vi "Lab Panel V6.00.vi"() -> ()   [LabVIEW 2017] (continued)
              n212 = call "sub vi-open serial port v1.vi"("Select COM port"=w223) -> ("Error"=→"Com Port Status":bool, "LOOPS"=→"Com setup loops":i32, "VISA Com out"=→"VISA Com out":refnum<visa-resource-name>)  [unwired: 12 in]
            }
            frame #1 {
              n213 = for {
                N: 1 -> [_]
                w274 = TRUE
                n214 = local read "Temp Simulate"() -> (w230:bool)
                n215 = local write "Temp read loop"(0) -> ()
                n216 = case shown="True" w230 {
                  frame False {
                  }
                  frame True {
                    w276 = 20
                    n217 = local write "Ambient Volts"(2.92) -> ()
                    n218 = global write "Global display 3.vi" "Ref deg C"(w276) -> ()
                    n219 = local write "Ref deg C"(w276) -> ()
                  }
                }
                n220 = call "sub vi - GET ALL TEMP v7.vi"("LA01-EN"=w274, "LA02-EN"=w274, "LA03-EN"=w274, "LA04-EN"=w274, "LA05-EN"=w274, "simulate"=w230, "Gen Cal Value"=1) -> ("ID"=w236:T29, "LA01 TEMP"=w272:T30, "LA02 TEMP"=w265:T30, "LA04 TEMP"=w251:T30, "LA03 TEMP"=w258:T30, "LA05 TEMP"=w244:T30)  [unwired: 3 in, 4 out]
                n221 = local write "LAB05 TEMP"(w244) -> ()
                n222 = local write "LAB04 TEMP"(w251) -> ()
                n223 = Unbundle(w258) -> ("T1"=w255:dbl, "T2"=w254:dbl, "T3"=w253:dbl, "T4"=w252:dbl)  [unwired: 2 out]
                n224 = Unbundle(w272) -> ("T1"=w270:dbl, "T2"=w269:dbl, "T3"=w268:dbl, "T4"=w267:dbl)  [unwired: 2 out]
                n225 = Unbundle(w265) -> ("T1"=w262:dbl, "T2"=w261:dbl, "T3"=w260:dbl, "T4"=w259:dbl)  [unwired: 2 out]
                n226 = Unbundle(w251) -> ("T1"=w249:dbl, "T2"=w248:dbl, "T3"=w247:dbl, "T4"=w246:dbl)  [unwired: 2 out]
                n227 = Unbundle(w244) -> ("T1"=w242:dbl, "T2"=w241:dbl, "T3"=w240:dbl, "T4"=w239:dbl)  [unwired: 2 out]
                n228 = local write "LAB01 TEMP"(w272) -> ()
                n229 = local write "LAB02 TEMP"(w265) -> ()
                n230 = local write "LAB03 TEMP"(w258) -> ()
                n231 = Unbundle(w236) -> ("id1"=→"LAB01-TP":bool, "id2"=→"LAB02-TP":bool, "id3"=→"LAB03-TP":bool, "id4"=→"LAB04-TP":bool, "id5"=→"LAB05-TP":bool)
                n232 = local read "TEMP LA05"() -> (w243:T9)
                n233 = local read "TEMP LA04"() -> (w250:T9)
                n234 = local read "TEMP LA02"() -> (w264:T9)
                n235 = local read "TEMP LA03"() -> (w257:T9)
                n236 = local read "TEMP LA01"() -> (w271:T9)
                n237 = Bundle(cluster=w257, "TL-1"=w255, "TN-1"=w254, "TL-2"=w253, "TN-2"=w252) -> (w256:T9)  [unwired: 4 in]
                n238 = Bundle(cluster=w271, "TL-1"=w270, "TN-1"=w269, "TL-2"=w268, "TN-2"=w267) -> (w266:T9)  [unwired: 4 in]
                n239 = Bundle(cluster=w264, "TL-1"=w262, "TN-1"=w261, "TL-2"=w260, "TN-2"=w259) -> (w263:T9)  [unwired: 4 in]
                n240 = Bundle(cluster=w250, "TL-1"=w249, "TN-1"=w248, "TL-2"=w247, "TN-2"=w246) -> (w245:T9)  [unwired: 4 in]
                n241 = Bundle(cluster=w243, "TL-1"=w242, "TN-1"=w241, "TL-2"=w240, "TN-2"=w239) -> (w238:T9)  [unwired: 4 in]
                n242 = local write "TEMP LA03"(w256) -> ()
                n243 = local write "TEMP LA01"(w266) -> ()
                n244 = local write "TEMP LA02"(w263) -> ()
                n245 = local write "TEMP LA05"(w238) -> ()
                n246 = local write "TEMP LA04"(w245) -> ()
              }
            }
            frame #2 {
              w285 = 0
              n247 = local read "LAB01 TEMP"() -> (w287:T12)
              n248 = local read "SIG LAB01-2"() -> (w282:T2)
              n249 = Unbundle By Name(w287) -> ("T1 Live"=w280:dbl, "T1 Neut"=w279:dbl, "T2 Live"=w278:dbl, "T2 Neut"=w277:dbl)  [unwired: 2 out]
              n250 = local read "SIG LAB01-1"() -> (w284:T2)
              n251 = local read "TEMP LA01"() -> (w288:T9)
              n252 = Bundle By Name(cluster=w288, "TL-1"=w280, "TN-1"=w279, "TL-2"=w278, "TN-2"=w277, "TL -1COUNT"=w285, "TN-1 COUNT"=w285, "TL-2 COUNT"=w285, "TN-2 COUNT"=w285) -> (w286:T9)
              n253 = Bundle(cluster=w284, "Tmp Live"=w280, "Tmp Neut"=w279) -> (w283:T2)  [unwired: 3 in]
              n254 = Bundle(cluster=w282, "Tmp Live"=w278, "Tmp Neut"=w277) -> (w281:T2)  [unwired: 3 in]
              n255 = local write "SIG LAB01-2"(w281) -> ()
              n256 = local write "SIG LAB01-1"(w283) -> ()
              n257 = local write "TEMP LA01"(w286) -> ()
            }
            frame #3 {
              w297 = 0
              n258 = local read "LAB02 TEMP"() -> (w299:T12)
              n259 = Unbundle By Name(w299) -> ("T1 Live"=w292:dbl, "T1 Neut"=w291:dbl, "T2 Live"=w290:dbl, "T2 Neut"=w289:dbl)  [unwired: 2 out]
              n260 = local read "SIG LAB02-1"() -> (w296:T2)
              n261 = local read "SIG LAB02-2"() -> (w295:T2)
              n262 = local read "TEMP LA02"() -> (w300:T9)
              n263 = Bundle By Name(cluster=w300, "TL-1"=w292, "TN-1"=w291, "TL-2"=w290, "TN-2"=w289, "TL -1COUNT"=w297, "TN-1 COUNT"=w297, "TL-2 COUNT"=w297, "TN-2 COUNT"=w297) -> (w298:T9)
              n264 = Bundle(cluster=w295, "Tmp Live"=w290, "Tmp Neut"=w289) -> (w293:T2)  [unwired: 3 in]
              n265 = Bundle(cluster=w296, "Tmp Live"=w292, "Tmp Neut"=w291) -> (w294:T2)  [unwired: 3 in]
              n266 = local write "TEMP LA02"(w298) -> ()
              n267 = local write "SIG LAB02-1"(w294) -> ()
              n268 = local write "SIG LAB02-2"(w293) -> ()
            }
            frame #4 {
              w309 = 0
              n269 = local read "LAB03 TEMP"() -> (w311:T12)
              n270 = Unbundle By Name(w311) -> ("T1 Live"=w304:dbl, "T1 Neut"=w303:dbl, "T2 Live"=w302:dbl, "T2 Neut"=w301:dbl)  [unwired: 2 out]
              n271 = local read "SIG LAB03-1"() -> (w308:T2)
              n272 = local read "SIG LAB03-2"() -> (w307:T2)
              n273 = local read "TEMP LA03"() -> (w312:T9)
              n274 = Bundle By Name(cluster=w312, "TL-1"=w304, "TN-1"=w303, "TL-2"=w302, "TN-2"=w301, "TL -1COUNT"=w309, "TN-1 COUNT"=w309, "TL-2 COUNT"=w309, "TN-2 COUNT"=w309) -> (w310:T9)
              n275 = Bundle(cluster=w307, "Tmp Live"=w302, "Tmp Neut"=w301) -> (w305:T2)  [unwired: 3 in]
              n276 = Bundle(cluster=w308, "Tmp Live"=w304, "Tmp Neut"=w303) -> (w306:T2)  [unwired: 3 in]
              n277 = local write "TEMP LA03"(w310) -> ()
              n278 = local write "SIG LAB03-2"(w305) -> ()
              n279 = local write "SIG LAB03-1"(w306) -> ()
            }
            frame #5 {
              w321 = 0
              n280 = local read "LAB04 TEMP"() -> (w323:T12)
              n281 = Unbundle By Name(w323) -> ("T1 Live"=w316:dbl, "T1 Neut"=w315:dbl, "T2 Live"=w314:dbl, "T2 Neut"=w313:dbl)  [unwired: 2 out]
              n282 = local read "SIG LAB04-2"() -> (w319:T2)
              n283 = local read "SIG LAB04-1"() -> (w320:T2)
              n284 = local read "TEMP LA04"() -> (w324:T9)
              n285 = Bundle By Name(cluster=w324, "TL-1"=w316, "TN-1"=w315, "TL-2"=w314, "TN-2"=w313, "TL -1COUNT"=w321, "TN-1 COUNT"=w321, "TL-2 COUNT"=w321, "TN-2 COUNT"=w321) -> (w322:T9)
              n286 = Bundle(cluster=w319, "Tmp Live"=w314, "Tmp Neut"=w313) -> (w317:T2)  [unwired: 3 in]
              n287 = Bundle(cluster=w320, "Tmp Live"=w316, "Tmp Neut"=w315) -> (w318:T2)  [unwired: 3 in]
              n288 = local write "SIG LAB04-2"(w317) -> ()
              n289 = local write "TEMP LA04"(w322) -> ()
              n290 = local write "SIG LAB04-1"(w318) -> ()
            }
            frame #6 {
              w333 = 0
              n291 = local read "LAB05 TEMP"() -> (w335:T12)
              n292 = Unbundle By Name(w335) -> ("T1 Live"=w328:dbl, "T1 Neut"=w327:dbl, "T2 Live"=w326:dbl, "T2 Neut"=w325:dbl)  [unwired: 2 out]
              n293 = local read "SIG LAB05-2"() -> (w331:T2)
              n294 = local read "SIG LAB05-1"() -> (w332:T2)
              n295 = local read "TEMP LA05"() -> (w336:T9)
              n296 = Bundle By Name(cluster=w336, "TL-1"=w328, "TN-1"=w327, "TL-2"=w326, "TN-2"=w325, "TL -1COUNT"=w333, "TN-1 COUNT"=w333, "TL-2 COUNT"=w333, "TN-2 COUNT"=w333) -> (w334:T9)
              n297 = Bundle(cluster=w331, "Tmp Live"=w326, "Tmp Neut"=w325) -> (w329:T2)  [unwired: 3 in]
              n298 = Bundle(cluster=w332, "Tmp Live"=w328, "Tmp Neut"=w327) -> (w330:T2)  [unwired: 3 in]
              n299 = local write "SIG LAB05-2"(w329) -> ()
              n300 = local write "SIG LAB05-1"(w330) -> ()
              n301 = local write "TEMP LA05"(w334) -> ()
            }
          }
        }
        frame #11 {
          # "Create analog task"
          n302 = local read "DAQ Simulate"() -> (w338:bool)
          n303 = case shown="False" w338 {
            tunnel: w337 -> [w340 _]
            frame False {
              n304 = local read "RATE (Hz)"() -> (w347:dbl)
              n305 = local read "SAMPLES"() -> (w346:dbl)
              n306 = call "sub vi - AI USB4704 (3)  Create Task v4.vi"("Test"=w340, "Rate Hz"=w347, "Samples"=w346) -> ("physical channels 0"=→"physical channels 0":string, "physical channels 1"=→"physical channels 1":string, "physical channels 2"=→"physical channels 2":string, "TASK USB 0"=→"AI Task0":i32, "TASK USB 1"=→"AI Task1":i32, "TASK USB 2"=→"AI Task2":i32, "AI Task Er"=w344:bool, "error array"=→"error array":errorcluster[])  [unwired: 5 in]
              n307 = local write "Reset Error"(w344) -> ()
              "AI Task" <- TRUE
            }
            frame True {
            }
          }
        }
        frame #12 {
          # "Enable front panel, all settings done"
          n308 = property on="Tab Control 2" class="TabCtl (strict)"("DisabledEnum"=T18."Enabled" ("Disabled")) -> ()  [unwired: 2 in, 2 out]
          n309 = property on="Tab Control 2" class="TabCtl (strict)"("Value"=0) -> ()  [unwired: 2 in, 2 out]
        }
        frame #13 {
          n310 = property on="Tab Control 2" class="TabCtl (strict)"("Value"=0) -> ()  [unwired: 2 in, 2 out]
        }
      }
    }
    frame #2 {
      # "frames that only action on certain cycles, 13, 14, 15, 16, 19, 21"
      # "Main Loop"
      n311 = node-c288("Set Loop Time") -> (w357:T20)  [unwired: 3 in]
      n312 = timed-loop {
        timing: w357 -> [_]
        timing-out: [_] -> w356
        tunnel: "Set Loop Time" -> [w360]
        tunnel: w354 -> [w359]
        i -> [w386]
        stop <- w361 stop-if-true
        n313 = node-c288() -> (→"Timed loop Finished Late":bool)  [unwired: 1 in, 4 out]
        n314 = local read "Resets Done"() -> (w365:dbl)
        n315 = local read "SELECT LAB05-2"() -> (w366:T3)
        n316 = local read "SELECT LAB05-1"() -> (w367:T3)
        n317 = local read "SELECT LAB04-2"() -> (w368:T3)
        n318 = local read "SELECT LAB03-1"() -> (w371:T3)
        n319 = local read "SELECT LAB02-2"() -> (w372:T3)
        n320 = local read "SELECT LAB03-2"() -> (w370:T3)
        n321 = local read "SELECT LAB04-1"() -> (w369:T3)
        n322 = local read "SELECT LAB02-1"() -> (w373:T3)
        n323 = local read "run lab03-2"() -> (w380:bool)
        n324 = local read "run lab04-1"() -> (w379:bool)
        n325 = local read "run lab05-1"() -> (w377:bool)
        n326 = local read "run lab04-2"() -> (w378:bool)
        n327 = local read "run lab05-2"() -> (w376:bool)
        n328 = local read "run lab03-1"() -> (w381:bool)
        n329 = local read "run lab02-2"() -> (w382:bool)
        n330 = local read "SELECT LAB01-1"() -> (w375:T3)
        n331 = local read "SELECT LAB01-2"() -> (w374:T3)
        n332 = local read "run lab02-1"() -> (w383:bool)
        n333 = Greater?(x=w365, y=50) -> (0:w362:bool)
        n334 = Or(x=w362, y="stop") -> (x .or. y?=w361:bool)
        n335 = local read "run lab01-1"() -> (w385:bool)
        n336 = local read "run lab01-2"() -> (w384:bool)
        n337 = global write "Global display 1.vi" "stop disp"(w361) -> ()
        n338 = stacked-sequence {
          seq-local: [_ _ w508 _ _ _ _ _ _ _ _ _ _ _ _ _ _ _ _ _ _ _ _ _ _ _ _] -> [_ _ _ _ _ _ w2614 _ _ _ _ _ _ _ _ _ _ _ _ _ _ _ _ _ _ _ _]
          seq-local: [_ _ w507 _ _ _ _ _ _ _ _ _ _ _ _ _ _ _ _ _ _ _ _ _ _ _ _] -> [_ _ _ _ _ _ w2613 _ _ _ _ _ _ _ _ _ _ _ _ _ _ _ _ _ _ _ _]
          seq-local: [_ _ w494 _ _ _ _ _ _ _ _ _ _ _ _ _ _ _ _ _ _ _ _ _ _ _ _] -> [_ _ _ _ _ _ w2612 _ _ _ _ _ _ _ _ _ _ _ _ _ _ _ _ _ _ _ _]
          seq-local: [_ _ w493 _ _ _ _ _ _ _ _ _ _ _ _ _ _ _ _ _ _ _ _ _ _ _ _] -> [_ _ _ _ _ _ w2611 _ _ _ _ _ _ _ _ _ _ _ _ _ _ _ _ _ _ _ _]
          seq-local: [_ _ w492 _ _ _ _ _ _ _ _ _ _ _ _ _ _ _ _ _ _ _ _ _ _ _ _] -> [_ _ _ _ _ _ w2610 _ _ _ _ _ _ _ _ _ _ _ _ _ _ _ _ _ _ _ _]
          seq-local: [_ _ w491 _ _ _ _ _ _ _ _ _ _ _ _ _ _ _ _ _ _ _ _ _ _ _ _] -> [_ _ _ _ _ _ w2609 _ _ _ _ _ _ _ _ _ _ _ _ _ _ _ _ _ _ _ _]
          seq-local: [_ _ w490 _ _ _ _ _ _ _ _ _ _ _ _ _ _ _ _ _ _ _ _ _ _ _ _] -> [_ _ _ _ _ _ w2608 _ _ _ _ _ _ _ _ _ _ _ _ _ _ _ _ _ _ _ _]
          seq-local: [_ _ w489 _ _ _ _ _ _ _ _ _ _ _ _ _ _ _ _ _ _ _ _ _ _ _ _] -> [_ _ _ _ _ _ w2607 _ _ _ _ _ _ _ _ _ _ _ _ _ _ _ _ _ _ _ _]
          seq-local: [_ _ w488 _ _ _ _ _ _ _ _ _ _ _ _ _ _ _ _ _ _ _ _ _ _ _ _] -> [_ _ _ _ _ _ w2606 _ _ _ _ _ _ _ _ _ _ _ _ _ _ _ _ _ _ _ _]
          seq-local: [_ _ w487 _ _ _ _ _ _ _ _ _ _ _ _ _ _ _ _ _ _ _ _ _ _ _ _] -> [_ _ _ _ _ _ w2605 _ _ _ _ _ _ _ _ _ _ _ _ _ _ _ _ _ _ _ _]
          seq-local: [_ _ _ _ _ _ _ _ _ _ _ _ w3809 _ _ _ _ _ _ _ _ _ _ _ _ _ _] -> [_ _ _ _ _ _ _ _ _ _ _ _ _ w3846 _ _ _ _ _ _ _ _ _ _ _ _ _]
          seq-local: [w391 _ _ _ _ _ _ _ _ _ _ _ _ _ _ _ _ _ _ _ _ _ _ _ _ _ _] -> [_ _ _ _ _ _ _ _ _ _ _ _ _ _ _ _ _ _ _ _ _ _ _ _ _ _ w6562]
          tunnel: w385 -> [_ _ _ w525 w777 w2204 w2634 w2950 w3438 _ _ _ _ _ w4163 _ w5121 _ _ w5472 w5776 w5957 _ _ _ _ _]
          tunnel: w384 -> [_ _ _ w524 w775 w2203 w2633 w2951 w3437 _ _ _ _ _ w4162 _ w5119 _ _ w5471 w5775 w5955 _ _ _ _ _]
          tunnel: w383 -> [_ _ _ w523 w773 w2202 w2632 w2949 w3436 _ _ _ _ _ w4161 _ w5117 _ _ w5470 w5774 w5954 _ _ _ _ _]
          tunnel: w382 -> [_ _ _ w522 w771 w2201 w2631 w2948 w3435 _ _ _ _ _ w4160 _ w5115 _ _ w5469 w5773 w5953 _ _ _ _ _]
          tunnel: w381 -> [_ _ _ w521 w769 w2200 w2630 w2947 w3434 _ _ _ _ _ w4159 _ w5113 _ _ w5468 w5772 w5952 _ _ _ _ _]
          tunnel: w380 -> [_ _ _ w520 w767 w2199 w2629 w2946 w3433 _ _ _ _ _ w4158 _ w5111 _ _ w5467 w5771 w5951 _ _ _ _ _]
          tunnel: w379 -> [_ _ _ w519 w765 w2198 w2628 w2945 w3432 _ _ _ _ _ w4157 _ w5109 _ _ w5466 w5770 w5950 _ _ _ _ _]
          tunnel: w378 -> [_ _ _ w518 w763 w2197 w2627 w2944 w3431 _ _ _ _ _ w4156 _ w5107 _ _ w5465 w5769 w5949 _ _ _ _ _]
          tunnel: w377 -> [_ _ _ w517 w761 w2196 w2626 w2943 w3430 _ _ _ _ _ w4155 _ w5105 _ _ w5464 w5768 w5948 _ _ _ _ _]
          tunnel: w376 -> [_ _ _ w516 w759 w2195 w2625 w2942 w3429 _ _ _ _ _ w4154 _ w5103 _ _ w5463 w5767 w5947 _ _ _ _ _]
          tunnel: w375 -> [_ _ _ _ w776 w2194 w2624 _ _ _ _ _ _ _ _ _ w5123 _ _ _ _ _ w6420 _ _ _ _]
          tunnel: w374 -> [_ _ _ _ w774 w2193 w2623 _ _ _ _ _ _ _ _ _ w5118 _ _ _ _ _ w6419 _ _ _ _]
          tunnel: w373 -> [_ _ _ _ w772 w2192 w2622 _ _ _ _ _ _ _ _ _ w5116 _ _ _ _ _ w6418 _ _ _ _]
          tunnel: w372 -> [_ _ _ _ w770 w2191 w2621 _ _ _ _ _ _ _ _ _ w5114 _ _ _ _ _ w6417 _ _ _ _]
          tunnel: w371 -> [_ _ _ _ w768 w2190 w2620 _ _ _ _ _ _ _ _ _ w5112 _ _ _ _ _ w6416 _ _ _ _]
          tunnel: w370 -> [_ _ _ _ w766 w2189 w2619 _ _ _ _ _ _ _ _ _ w5110 _ _ _ _ _ w6415 _ _ _ _]
          tunnel: w369 -> [_ _ _ _ w764 w2188 w2618 _ _ _ _ _ _ _ _ _ w5108 _ _ _ _ _ w6414 _ _ _ _]
          tunnel: w368 -> [_ _ _ _ w762 w2187 w2617 _ _ _ _ _ _ _ _ _ w5106 _ _ _ _ _ w6413 _ _ _ _]
          tunnel: w367 -> [_ _ _ _ w760 w2186 w2616 _ _ _ _ _ _ _ _ _ w5104 _ _ _ _ _ w6412 _ _ _ _]
          tunnel: w366 -> [_ _ _ _ w758 w2185 w2615 _ _ _ _ _ _ _ _ _ w5102 _ _ _ _ _ w6411 _ _ _ _]
          tunnel: w362 -> [_ _ _ _ _ _ _ _ _ _ _ _ _ _ _ _ _ _ _ _ _ _ _ _ w6523 _ _]
          tunnel: w361 -> [_ _ _ _ _ _ _ _ _ _ _ _ _ _ _ _ _ _ _ _ _ _ _ _ w6522 _ _]
          tunnel: w360 -> [_ w440 _ _ _ _ _ _ _ _ _ _ _ _ _ _ _ _ _ _ _ _ _ _ _ _ _]
          tunnel: w359 -> [w390 _ _ w511 _ _ _ _ _ _ _ w3605 w3807 _ _ _ _ _ _ _ _ _ _ _ _ _ _]
          frame #0 {
            # "Acquire analog Inputs"
            n339 = Tick Count (ms)() -> (millisecond timer value=w391:u32)
            n340 = global write "Global 1.vi" "RATE(Hz)"("RATE (Hz)") -> ()
            n341 = local read "AI Task"() -> (w393:bool)
            n342 = case shown="True" w393 {
              tunnel: "RATE (Hz)" -> [_ _]
              tunnel: w390 -> [_ w403]
              tunnel: w390 -> [_ w402]
              frame False {
              }
              frame True {
                n343 = Tick Count (ms)() -> (millisecond timer value=w407:u32)
                n344 = flat-sequence {
                  tunnel: w407 -> [w409]
                  tunnel: [w409] -> w406
                  tunnel: w403 -> [w408]
                  tunnel: w406 -> [w418]
                  tunnel: [w416] -> w404
                  tunnel: [w424] -> w405
                  tunnel: w404 -> [w424]
                  tunnel: w402 -> [w422]
                  tunnel: [w419] -> w401
                  tunnel: w405 -> [w436]
                  tunnel: w401 -> [w434]
                  frame #0 {
                    n345 = disable-structure shown="Disabled" {
                      disable-tunnel: w408 -> [w410 _]
                      frame Disabled {
                        n346 = local read "RATE (Hz)"() -> (w415:dbl)
                        n347 = local read "SAMPLES"() -> (w414:dbl)
                        n348 = call "sub vi - AI USB4704 (3)  Create Task v4.vi"("Test"=w410, "Rate Hz"=w415, "Samples"=w414) -> ("TASK USB 0"=w412:i32, "TASK USB 1"=w413:i32, "TASK USB 2"=w411:i32)  [unwired: 5 in, 5 out]
                        n349 = local write "AI Task0"(w412) -> ()
                        n350 = local write "AI Task1"(w413) -> ()
                        n351 = local write "AI Task2"(w411) -> ()
                      }
                      frame Enabled {
                      }
                    }
                  }
                  frame #1 {
                    n352 = Tick Count (ms)() -> (millisecond timer value=w416:u32)
                    n353 = Subtract(x=w416, y=w418) -> (x-y=→"ACQ Init TIme":u32)
                  }
                  frame #2 {
                    n354 = local read "SAMPLES"() -> (w425:dbl)
                    n355 = local read "AI Task0"() -> (w432:u64)
                    n356 = local read "AI Task1"() -> (w431:u32)
                    n357 = local read "AI Task2"() -> (w430:u32)
                    n358 = local read "MAIL SETTINGS"() -> (w423:T7)
                    n359 = call "sub vi - AI USB4704 (3) v73.vi"("Task0"=w432, "Test"=w422, "Task1"=w431, "Task2"=w430, "SAMPLES"=w425, "MAIL SETTINGS"=w423) -> ("Fault"=w419:bool, "data 0"=→"AI data 0" →"AI Data 0":waveform(dbl)[], "data 1"=→"AI data 1" →"AI Data 1":waveform(dbl)[], "data 2"=w420:waveform(dbl)[], "loop time"=→"AI loop time":dbl, "Fault Counts"=→"Analog Fault Counts":i32[], "error array"=→"AI Error":errorcluster[])  [unwired: 3 in]
                    "AI data 2" <- w420
                    "AI Data 2" <- w420
                    n360 = local write "Analog error"(w419) -> ()
                    n361 = disable-structure shown="Disabled" {
                      disable-tunnel: w420 -> [w433 _]
                      frame Disabled {
                        n362 = call "Save Analog Data.vi"("AI data 2"=w433) -> ()  [unwired: 11 in]
                      }
                      frame Enabled {
                      }
                    }
                  }
                  frame #3 {
                    n363 = Tick Count (ms)() -> (millisecond timer value=w437:u32)
                    n364 = Tick Count (ms)() -> ()  [unwired: 1 out]
                    n365 = case shown="True" w434 {
                      frame False {
                      }
                      frame True {
                        n366 = call "Less Simple Error Handler.vi"("message"="Ananlog error") -> ()  [unwired: 5 in]
                      }
                    }
                    n367 = Subtract(x=w437, y=w436) -> (x-y=→"ACQ Time":u32)
                  }
                }
              }
            }
            n368 = disable-structure shown="Disabled" {
              frame Disabled {
                n369 = call <userlib>:"Periodic Trigger__ogtk.vi"("time (ms)"=u32 1000) -> ("Triggered"=w395:bool)  [unwired: 12 in, 2 out]
                n370 = case shown="True" w395 {
                  frame False {
                  }
                  frame True {
                    n371 = control-ref of="This VI"() -> (w400:refnum<vi>)
                    n372 = invoke class="VI" method="FP.Get Image"(reference=w400) -> ("image data"=w399:T31)  [unwired: 5 in, 5 out]
                    n373 = Build Path(base path="path to JPEG file", name or relative path="FP.jpg") -> (appended path=w396:path)
                    n374 = call <vilib>:"Write JPEG File.vi"("image data"=w399, "path to JPEG file"=w396) -> ()  [unwired: 8 in, 2 out]
                  }
                }
              }
              frame Enabled {
              }
            }
          }
          frame #1 {
            w447 = FALSE
            # "Loop time (s)"
            # "set up cycle control"
            n375 = local read "jig cycle"() -> (w451:dbl)
            n376 = local read "Amps Fail level"() -> (w445:dbl)
            n377 = local read "DAQ Simulate"() -> (w442:bool)
            n378 = Divide(x=w440, y=1000.0) -> (x/y=w439:T14)
            n379 = Divide(x="JIG ON TIME (S)", y=w439) -> (x/y=→"on loops":T14)
            n380 = Divide(x="JIG OFF TIME (S)", y=w439) -> (x/y=→"off loops":T14)
            n381 = Increment(x=w451) -> (x+1=w450:dbl)
            n382 = local write "Simulate IND"(w442) -> ()
            n383 = global write "Global display 3.vi" "Amps Fail"(w445) -> ()
            n384 = local write "TEMP"(w447) -> ()
            n385 = local write "AI"(w447) -> ()
            n386 = local read "Network Directory"() -> (w444:path)
            n387 = local write "jig cycle"(w450) -> ()
            n388 = call "sub vi - check network dir v2.vi"("PATH"=w444) -> ("error"=w443:bool)  [unwired: 10 in]
            n389 = disable-structure shown="Enabled" {
              frame Enabled {
                n390 = property on="Tab Control 2" class="TabCtl (strict)"() -> ("Pages"=w455:refnum<vi>[])  [unwired: 2 in, 2 out]
                n391 = Index Array(array=w455, index=8) -> (element=w457:refnum<vi>)
                n392 = property class="Page"(reference=w457, "PageVis"=TRUE) -> ()  [unwired: 1 in, 2 out]
              }
              frame Disabled {
              }
            }
            n393 = global write "Global display 3.vi" "network drive"(w443) -> ()
            n394 = event shown="[1] \"ADMIN\": Value Change" {
              selector: _ -> [_ _]
              dyn-events: _ -> [_ _]
              timeout: 10 -> [_ _]
              event Timeout {
                n395 = event-data() -> ()  [unwired: 1 in, 3 out]
              }
              event "ADMIN": Value Change {
                n396 = event-data() -> ()  [unwired: 1 in, 6 out]
                n397 = stacked-sequence {
                  seq-local: [_ w459 _] -> [_ _ w460]
                  frame #0 {
                    n398 = global write "Global 1.vi" "password"("9949") -> ()
                  }
                  frame #1 {
                    n399 = call "sub vi - password 1.vi"() -> ("RESULT"=w459:bool)  [unwired: 11 in]
                  }
                  frame #2 {
                    w462 = FALSE
                    n400 = property on="Tab Control 2" class="TabCtl (strict)"() -> ("Pages"=w466:refnum<vi>[])  [unwired: 2 in, 2 out]
                    n401 = Select(t=TRUE, s=w460, f=w462) -> (s? t:f=w461:bool)
                    n402 = Index Array(array=w466, index=8) -> (element=w464:refnum<vi>)
                    n403 = property class="Page"(reference=w464, "PageVis"=w461) -> ()  [unwired: 1 in, 2 out]
                    n404 = local write "ADMIN"(w462) -> ()
                  }
                }
              }
            }
            n405 = local write "network error"(w443) -> ()
          }
          frame #2 {
            w504 = 60.0
            # "Test Cycles"
            # "seconds"
            # "convert temperature rise minutes to cycles"
            n406 = local read "SET LAB05-2"() -> (w468:T5)
            n407 = local read "SET LAB05-1"() -> (w470:T5)
            n408 = local read "SET LAB04-2"() -> (w472:T5)
            n409 = local read "SET LAB01-1"() -> (w486:T5)
            n410 = local read "SET LAB01-2"() -> (w484:T5)
            n411 = local read "SET LAB02-2"() -> (w480:T5)
            n412 = local read "SET LAB04-1"() -> (w474:T5)
            n413 = local read "SET LAB03-1"() -> (w478:T5)
            n414 = local read "SET LAB03-2"() -> (w476:T5)
            n415 = local read "SET LAB02-1"() -> (w482:T5)
            n416 = local read "JIG OFF TIME (S)"() -> (w509:dbl)
            n417 = local read "JIG ON TIME (S)"() -> (w510:dbl)
            n418 = Unbundle By Name(w486) -> ("T-RISE mins"=w485:dbl)
            n419 = Unbundle(w468) -> ("T-RISE mins"=w467:dbl)  [unwired: 4 out]
            n420 = Unbundle(w470) -> ("T-RISE mins"=w469:dbl)  [unwired: 4 out]
            n421 = Unbundle(w472) -> ("T-RISE mins"=w471:dbl)  [unwired: 4 out]
            n422 = Unbundle(w484) -> ("T-RISE mins"=w483:dbl)  [unwired: 4 out]
            n423 = Unbundle(w482) -> ("T-RISE mins"=w481:dbl)  [unwired: 4 out]
            n424 = Unbundle(w474) -> ("T-RISE mins"=w473:dbl)  [unwired: 4 out]
            n425 = Unbundle(w480) -> ("T-RISE mins"=w479:dbl)  [unwired: 4 out]
            n426 = Unbundle(w476) -> ("T-RISE mins"=w475:dbl)  [unwired: 4 out]
            n427 = Unbundle(w478) -> ("T-RISE mins"=w477:dbl)  [unwired: 4 out]
            n428 = Add(x=w510, y=w509) -> (x+y=w503:dbl)
            n429 = Multiply(x=w504, y=w475) -> (x*y=w499:dbl)
            n430 = Multiply(x=w504, y=w473) -> (x*y=w498:dbl)
            n431 = Multiply(x=w504, y=w471) -> (x*y=w497:dbl)
            n432 = Multiply(x=w504, y=w469) -> (x*y=w496:dbl)
            n433 = Multiply(x=w504, y=w467) -> (x*y=w495:dbl)
            n434 = Multiply(x=w504, y=w483) -> (x*y=w505:dbl)
            n435 = Multiply(x=w504, y=w477) -> (x*y=w500:dbl)
            n436 = Multiply(x=w504, y=w485) -> (x*y=w506:dbl)
            n437 = Multiply(x=w504, y=w481) -> (x*y=w502:dbl)
            n438 = Multiply(x=w504, y=w479) -> (x*y=w501:dbl)
            n439 = Divide(x=w496, y=w503) -> (x/y=w488:dbl)
            n440 = Divide(x=w497, y=w503) -> (x/y=w489:dbl)
            n441 = Divide(x=w498, y=w503) -> (x/y=w490:dbl)
            n442 = Divide(x=w495, y=w503) -> (x/y=w487:dbl)
            n443 = Divide(x=w500, y=w503) -> (x/y=w492:dbl)
            n444 = Divide(x=w506, y=w503) -> (x/y=w508:dbl)
            n445 = Divide(x=w505, y=w503) -> (x/y=w507:dbl)
            n446 = Divide(x=w502, y=w503) -> (x/y=w494:dbl)
            n447 = Divide(x=w501, y=w503) -> (x/y=w493:dbl)
            n448 = Divide(x=w499, y=w503) -> (x/y=w491:dbl)
          }
          frame #3 {
            # "control cycle loops"
            n449 = local read "JIG OFF TIME (S)"() -> (w514:dbl)
            n450 = local read "JIG ON TIME (S)"() -> (w513:dbl)
            n451 = local read "on loops"() -> (w529:dbl)
            n452 = local read "off loops"() -> (w528:dbl)
            n453 = local read "jig cycle"() -> (w527:dbl)
            n454 = Add(x=w514, y=w513) -> (x+y=w512:dbl)
            n455 = Add(x=w529, y=w528) -> (x+y=w515:dbl)
            n456 = Greater Or Equal?(x=w527, y=w515) -> (x >= y?=w526:bool)
            n457 = case shown="True" w526 {
              tunnel: w525 -> [_ w564]
              tunnel: w524 -> [_ w563]
              tunnel: w523 -> [_ w562]
              tunnel: w522 -> [_ w561]
              tunnel: w521 -> [_ w560]
              tunnel: w520 -> [_ w559]
              tunnel: w519 -> [_ w558]
              tunnel: w518 -> [_ w557]
              tunnel: w517 -> [_ w556]
              tunnel: w516 -> [_ w555]
              tunnel: w512 -> [_ w554]
              tunnel: w511 -> [_ w530]
              frame False {
              }
              frame True {
                # "increment cycle value and convert cycles to minutes for temp rise"
                n458 = stacked-sequence {
                  tunnel: w530 -> [_ w568]
                  frame #0 {
                    n459 = local read "Temp read loop"() -> (w567:dbl)
                    n460 = Increment(x=w567) -> (x+1=w566:dbl)
                    n461 = local write "Temp read loop"(w566) -> ()
                  }
                  frame #1 {
                    n462 = case shown="True" w568 {
                      tunnel: [20 2] -> w570
                      frame False {
                      }
                      frame True {
                      }
                    }
                    n463 = local read "Temp read loop"() -> (w569:dbl)
                    n464 = Greater?(x=w569, y=w570) -> (0:w571:bool)
                    n465 = case shown="True" w571 {
                      frame False {
                      }
                      frame True {
                        n466 = local write "Temp read loop"(1) -> ()
                      }
                    }
                  }
                }
                n467 = local read "JIG RELAY CYCLES"() -> (w553:T8)
                n468 = local read "Temp read loop"() -> (→"Temp Up":dbl)
                n469 = Unbundle By Name(w553) -> ("LAB01-1"=w551:dbl, "LAB01-2"=w549:dbl, "LAB02-1"=w547:dbl, "LAB02-2"=w545:dbl, "LAB03-1"=w543:dbl, "LAB03-2"=w541:dbl, "LAB04-1"=w539:dbl, "LAB04-2"=w537:dbl, "LAB05-1"=w535:dbl, "LAB05-2"=w533:dbl)
                n470 = stacked-sequence {
                  tunnel: w564 -> [w585 _ _ _ _ _ _ _ _ _]
                  tunnel: w563 -> [_ w602 _ _ _ _ _ _ _ _]
                  tunnel: w562 -> [_ _ w619 _ _ _ _ _ _ _]
                  tunnel: w561 -> [_ _ _ w636 _ _ _ _ _ _]
                  tunnel: w560 -> [_ _ _ _ w653 _ _ _ _ _]
                  tunnel: w559 -> [_ _ _ _ _ w670 _ _ _ _]
                  tunnel: w558 -> [_ _ _ _ _ _ w687 _ _ _]
                  tunnel: w557 -> [_ _ _ _ _ _ _ w704 _ _]
                  tunnel: w556 -> [_ _ _ _ _ _ _ _ w721 _]
                  tunnel: w555 -> [_ _ _ _ _ _ _ _ _ w738]
                  tunnel: w554 -> [w582 w599 w616 w633 w650 w667 w684 w701 w718 w735]
                  tunnel: w551 -> [w576 _ _ _ _ _ _ _ _ _]
                  tunnel: [w575 _ _ _ _ _ _ _ _ _] -> w550
                  tunnel: w549 -> [_ w593 _ _ _ _ _ _ _ _]
                  tunnel: [_ w592 _ _ _ _ _ _ _ _] -> w548
                  tunnel: w547 -> [_ _ w610 _ _ _ _ _ _ _]
                  tunnel: [_ _ w609 _ _ _ _ _ _ _] -> w546
                  tunnel: w545 -> [_ _ _ w627 _ _ _ _ _ _]
                  tunnel: [_ _ _ w626 _ _ _ _ _ _] -> w544
                  tunnel: w543 -> [_ _ _ _ w644 _ _ _ _ _]
                  tunnel: [_ _ _ _ w643 _ _ _ _ _] -> w542
                  tunnel: w541 -> [_ _ _ _ _ w661 _ _ _ _]
                  tunnel: [_ _ _ _ _ w660 _ _ _ _] -> w540
                  tunnel: w539 -> [_ _ _ _ _ _ w678 _ _ _]
                  tunnel: [_ _ _ _ _ _ w677 _ _ _] -> w538
                  tunnel: w537 -> [_ _ _ _ _ _ _ w695 _ _]
                  tunnel: [_ _ _ _ _ _ _ w694 _ _] -> w536
                  tunnel: w535 -> [_ _ _ _ _ _ _ _ w712 _]
                  tunnel: [_ _ _ _ _ _ _ _ w711 _] -> w534
                  tunnel: w533 -> [_ _ _ _ _ _ _ _ _ w729]
                  tunnel: [_ _ _ _ _ _ _ _ _ w728] -> w532
                  frame #0 {
                    n471 = local read "DISP LAB01-1"() -> (w580:T4)
                    n472 = Unbundle By Name(w580) -> ("CYCLE"=w581:dbl)
                    n473 = case shown="True" w585 {
                      tunnel: w581 -> [w587 w591]
                      tunnel: [w587 w590] -> w579
                      tunnel: w576 -> [w586 w589]
                      tunnel: [w586 w588] -> w575
                      frame False {
                      }
                      frame True {
                        n474 = Increment(x=w589) -> (x+1=w588:dbl)
                        n475 = Increment(x=w591) -> (x+1=w590:dbl)
                      }
                    }
                    n476 = Multiply(x=w579, y=w582) -> (x*y=w583:dbl)
                    n477 = Divide(x=w583, y=60.0) -> (x/y=w578:dbl)
                    n478 = Bundle By Name(cluster=w580, "CYCLE"=w579, "MINS"=w578) -> (w577:T4)
                    n479 = local write "DISP LAB01-1"(w577) -> ()
                  }
                  frame #1 {
                    n480 = local read "DISP LAB01-2"() -> (w597:T4)
                    n481 = Unbundle By Name(w597) -> ("CYCLE"=w598:dbl)
                    n482 = case shown="True" w602 {
                      tunnel: w598 -> [w604 w608]
                      tunnel: [w604 w607] -> w595
                      tunnel: w593 -> [w603 w606]
                      tunnel: [w603 w605] -> w592
                      frame False {
                      }
                      frame True {
                        n483 = Increment(x=w606) -> (x+1=w605:dbl)
                        n484 = Increment(x=w608) -> (x+1=w607:dbl)
                      }
                    }
                    n485 = Multiply(x=w595, y=w599) -> (x*y=w600:dbl)
                    n486 = Divide(x=w600, y=60.0) -> (x/y=w594:dbl)
                    n487 = Bundle By Name(cluster=w597, "CYCLE"=w595, "MINS"=w594) -> (w596:T4)
                    n488 = local write "DISP LAB01-2"(w596) -> ()
                  }
                  frame #2 {
                    n489 = local read "DISP LAB02-1"() -> (w614:T4)
                    n490 = Unbundle By Name(w614) -> ("CYCLE"=w615:dbl)
                    n491 = case shown="True" w619 {
                      tunnel: [w621 w625] -> w612
                      tunnel: w615 -> [w621 w624]
                      tunnel: w610 -> [w620 w623]
                      tunnel: [w620 w622] -> w609
                      frame False {
                      }
                      frame True {
                        n492 = Increment(x=w623) -> (x+1=w622:dbl)
                        n493 = Increment(x=w624) -> (x+1=w625:dbl)
                      }
                    }
                    n494 = Multiply(x=w612, y=w616) -> (x*y=w617:dbl)
                    n495 = Divide(x=w617, y=60.0) -> (x/y=w611:dbl)
                    n496 = Bundle By Name(cluster=w614, "CYCLE"=w612, "MINS"=w611) -> (w613:T4)
                    n497 = local write "DISP LAB02-1"(w613) -> ()
                  }
                  frame #3 {
                    n498 = local read "DISP LAB02-2"() -> (w631:T4)
                    n499 = Unbundle By Name(w631) -> ("CYCLE"=w632:dbl)
                    n500 = case shown="True" w636 {
                      tunnel: [w638 w642] -> w630
                      tunnel: w632 -> [w638 w641]
                      tunnel: w627 -> [w637 w640]
                      tunnel: [w637 w639] -> w626
                      frame False {
                      }
                      frame True {
                        n501 = Increment(x=w640) -> (x+1=w639:dbl)
                        n502 = Increment(x=w641) -> (x+1=w642:dbl)
                      }
                    }
                    n503 = Multiply(x=w630, y=w633) -> (x*y=w634:dbl)
                    n504 = Divide(x=w634, y=60.0) -> (x/y=w629:dbl)
                    n505 = Bundle By Name(cluster=w631, "CYCLE"=w630, "MINS"=w629) -> (w628:T4)
                    n506 = local write "DISP LAB02-2"(w628) -> ()
                  }
                  frame #4 {
                    n507 = local read "DISP LAB03-1"() -> (w648:T4)
                    n508 = Unbundle(w648) -> ("CYCLE"=w649:dbl)  [unwired: 2 out]
                    n509 = case shown="True" w653 {
                      tunnel: [w655 w659] -> w645
                      tunnel: w649 -> [w655 w658]
                      tunnel: w644 -> [w654 w657]
                      tunnel: [w654 w656] -> w643
                      frame False {
                      }
                      frame True {
                        n510 = Increment(x=w657) -> (x+1=w656:dbl)
                        n511 = Increment(x=w658) -> (x+1=w659:dbl)
                      }
                    }
                    n512 = Multiply(x=w645, y=w650) -> (x*y=w651:dbl)
                    n513 = Divide(x=w651, y=60.0) -> (x/y=w646:dbl)
                    n514 = Bundle(cluster=w648, "CYCLE"=w645, "MINS"=w646) -> (w647:T4)  [unwired: 1 in]
                    n515 = local write "DISP LAB03-1"(w647) -> ()
                  }
                  frame #5 {
                    n516 = local read "DISP LAB03-2"() -> (w665:T4)
                    n517 = Unbundle(w665) -> ("CYCLE"=w666:dbl)  [unwired: 2 out]
                    n518 = case shown="True" w670 {
                      tunnel: [w672 w676] -> w664
                      tunnel: w666 -> [w672 w675]
                      tunnel: w661 -> [w671 w674]
                      tunnel: [w671 w673] -> w660
                      frame False {
                      }
                      frame True {
                        n519 = Increment(x=w674) -> (x+1=w673:dbl)
                        n520 = Increment(x=w675) -> (x+1=w676:dbl)
                      }
                    }
                    n521 = Multiply(x=w664, y=w667) -> (x*y=w668:dbl)
                    n522 = Divide(x=w668, y=60.0) -> (x/y=w663:dbl)
                    n523 = Bundle(cluster=w665, "CYCLE"=w664, "MINS"=w663) -> (w662:T4)  [unwired: 1 in]
                    n524 = local write "DISP LAB03-2"(w662) -> ()
                  }
                  frame #6 {
                    n525 = local read "DISP LAB04-1"() -> (w682:T4)
                    n526 = Unbundle(w682) -> ("CYCLE"=w683:dbl)  [unwired: 2 out]
                    n527 = case shown="True" w687 {
                      tunnel: [w689 w693] -> w680
                      tunnel: w683 -> [w689 w692]
                      tunnel: w678 -> [w688 w691]
                      tunnel: [w688 w690] -> w677
                      frame False {
                      }
                      frame True {
                        n528 = Increment(x=w691) -> (x+1=w690:dbl)
                        n529 = Increment(x=w692) -> (x+1=w693:dbl)
                      }
                    }
                    n530 = Multiply(x=w680, y=w684) -> (x*y=w685:dbl)
                    n531 = Divide(x=w685, y=60.0) -> (x/y=w679:dbl)
                    n532 = Bundle(cluster=w682, "CYCLE"=w680, "MINS"=w679) -> (w681:T4)  [unwired: 1 in]
                    n533 = local write "DISP LAB04-1"(w681) -> ()
                  }
                  frame #7 {
                    n534 = local read "DISP LAB04-2"() -> (w699:T4)
                    n535 = Unbundle(w699) -> ("CYCLE"=w700:dbl)  [unwired: 2 out]
                    n536 = case shown="True" w704 {
                      tunnel: [w706 w710] -> w697
                      tunnel: w700 -> [w706 w709]
                      tunnel: w695 -> [w705 w708]
                      tunnel: [w705 w707] -> w694
                      frame False {
                      }
                      frame True {
                        n537 = Increment(x=w708) -> (x+1=w707:dbl)
                        n538 = Increment(x=w709) -> (x+1=w710:dbl)
                      }
                    }
                    n539 = Multiply(x=w697, y=w701) -> (x*y=w703:dbl)
                    n540 = Divide(x=w703, y=60.0) -> (x/y=w696:dbl)
                    n541 = Bundle(cluster=w699, "CYCLE"=w697, "MINS"=w696) -> (w698:T4)  [unwired: 1 in]
                    n542 = local write "DISP LAB04-2"(w698) -> ()
                  }
                  frame #8 {
                    n543 = local read "DISP LAB05-1"() -> (w716:T4)
                    n544 = Unbundle(w716) -> ("CYCLE"=w717:dbl)  [unwired: 2 out]
                    n545 = case shown="True" w721 {
                      tunnel: [w723 w727] -> w714
                      tunnel: w717 -> [w723 w726]
                      tunnel: w712 -> [w722 w725]
                      tunnel: [w722 w724] -> w711
                      frame False {
                      }
                      frame True {
                        n546 = Increment(x=w725) -> (x+1=w724:dbl)
                        n547 = Increment(x=w726) -> (x+1=w727:dbl)
                      }
                    }
                    n548 = Multiply(x=w714, y=w718) -> (x*y=w719:dbl)
                    n549 = Divide(x=w719, y=60.0) -> (x/y=w713:dbl)
                    n550 = Bundle(cluster=w716, "CYCLE"=w714, "MINS"=w713) -> (w715:T4)  [unwired: 1 in]
                    n551 = local write "DISP LAB05-1"(w715) -> ()
                  }
                  frame #9 {
                    n552 = local read "DISP LAB05-2"() -> (w734:T4)
                    n553 = Unbundle(w734) -> ("CYCLE"=w733:dbl)  [unwired: 2 out]
                    n554 = case shown="True" w738 {
                      tunnel: [w740 w744] -> w732
                      tunnel: w733 -> [w740 w743]
                      tunnel: w729 -> [w739 w742]
                      tunnel: [w739 w741] -> w728
                      frame False {
                      }
                      frame True {
                        n555 = Increment(x=w742) -> (x+1=w741:dbl)
                        n556 = Increment(x=w743) -> (x+1=w744:dbl)
                      }
                    }
                    n557 = Multiply(x=w732, y=w735) -> (x*y=w736:dbl)
                    n558 = Divide(x=w736, y=60.0) -> (x/y=w731:dbl)
                    n559 = Bundle(cluster=w734, "CYCLE"=w732, "MINS"=w731) -> (w730:T4)  [unwired: 1 in]
                    n560 = local write "DISP LAB05-2"(w730) -> ()
                  }
                }
                n561 = local write "jig cycle"(0) -> ()
                n562 = Bundle By Name(cluster=w553, "LAB01-1"=w550, "LAB01-2"=w548, "LAB02-1"=w546, "LAB02-2"=w544, "LAB03-1"=w542, "LAB03-2"=w540, "LAB04-1"=w538, "LAB04-2"=w536, "LAB05-1"=w534, "LAB05-2"=w532) -> (w552:T8)
                n563 = local write "JIG RELAY CYCLES"(w552) -> ()
              }
            }
          }
          frame #4 {
            # "Note : Run lab0X-N variables are set which are written to digital I/O in frame 11"
            # "Why are these here?"
            # "START & STOP test RUN switch change, start test if true and stop test if false"
            n564 = Get Date/Time In Seconds() -> (seconds since 1Jan1904=w756:timestamp)
            n565 = local read "C drive data root dir"() -> (w749:path)
            n566 = Format Date/Time String(time format string (%c)="%b\\%a%d", seconds (now)=w756) -> (date/time string=w780:string)  [unwired: 1 in]
            n567 = Format Date/Time String(time format string (%c)="%H%M", seconds (now)=w756) -> (date/time string=w778:string)  [unwired: 1 in]
            n568 = Format Date/Time String(time format string (%c)="LabPanel%Y", seconds (now)=w756) -> (date/time string=w755:string)  [unwired: 1 in]
            n569 = Path To String(path=w749) -> (string=w752:string)
            n570 = global write "Global 1.vi" "C drive root path"(w749) -> ()
            n571 = local read "Ref deg C"() -> (w745:dbl)
            n572 = Concatenate Strings(w752, "\\") -> (w750:string)
            n573 = event shown="[1] \"RUN LAB01-1\": Value Change" {
              selector: _ -> [_ _ _ _ _ _ _ _ _ _ _]
              dyn-events: _ -> [_ _ _ _ _ _ _ _ _ _ _]
              timeout: 10 -> [_ _ _ _ _ _ _ _ _ _ _]
              tunnel: w750 -> [_ w793 w933 w1074 w1214 w1354 w1494 w1634 w1774 w1914 w2055]
              tunnel: w780 -> [_ w792 w932 w1073 w1213 w1353 w1493 w1633 w1773 w1913 w2054]
              tunnel: w778 -> [_ w790 w931 w1072 w1212 w1352 w1492 w1632 w1772 w1912 w2053]
              tunnel: w776 -> [_ w791 _ _ _ _ _ _ _ _ _]
              tunnel: w777 -> [_ _ _ _ _ _ _ _ _ _ _]
              tunnel: w775 -> [_ _ _ _ _ _ _ _ _ _ _]
              tunnel: w774 -> [_ _ w930 _ _ _ _ _ _ _ _]
              tunnel: w773 -> [_ _ _ _ _ _ _ _ _ _ _]
              tunnel: w772 -> [_ _ _ w1071 _ _ _ _ _ _ _]
              tunnel: w771 -> [_ _ _ _ _ _ _ _ _ _ _]
              tunnel: w770 -> [_ _ _ _ w1211 _ _ _ _ _ _]
              tunnel: w769 -> [_ _ _ _ _ _ _ _ _ _ _]
              tunnel: w768 -> [_ _ _ _ _ w1351 _ _ _ _ _]
              tunnel: w767 -> [_ _ _ _ _ _ _ _ _ _ _]
              tunnel: w766 -> [_ _ _ _ _ _ w1491 _ _ _ _]
              tunnel: w765 -> [_ _ _ _ _ _ _ _ _ _ _]
              tunnel: w764 -> [_ _ _ _ _ _ _ w1631 _ _ _]
              tunnel: w763 -> [_ _ _ _ _ _ _ _ _ _ _]
              tunnel: w762 -> [_ _ _ _ _ _ _ _ w1771 _ _]
              tunnel: w761 -> [_ _ _ _ _ _ _ _ _ _ _]
              tunnel: w760 -> [_ _ _ _ _ _ _ _ _ w1911 _]
              tunnel: w759 -> [_ _ _ _ _ _ _ _ _ _ _]
              tunnel: w758 -> [_ _ _ _ _ _ _ _ _ _ w2052]
              tunnel: w755 -> [_ w789 w929 w1070 w1210 w1350 w1490 w1630 w1770 w1910 w2051]
              tunnel: [_ w788 w928 w1069 w1209 w1349 w1489 w1629 w1769 w1909 w2050] -> w753
              tunnel: "RESET CYCLES TO ZERO?" -> [_ w787 w926 w1067 w1207 w1347 w1487 w1627 w1767 w1907 w2048]
              tunnel: "YES" -> [_ w786 w925 w1066 w1206 w1346 w1486 w1626 w1766 w1906 w2047]
              tunnel: "NO" -> [_ w785 w924 w1065 w1205 w1345 w1485 w1625 w1765 w1905 w2046]
              tunnel: w745 -> [_ w782 w923 w1063 w1204 w1344 w1484 w1624 w1764 w1904 w2044]
              event Timeout {
                n574 = event-data() -> ()  [unwired: 1 in, 3 out]
              }
              event "RUN LAB01-1": Value Change {
                n575 = event-data() -> ("NewVal"=w783:bool)  [unwired: 1 in, 5 out]
                n576 = local read "SIG LAB01-1"() -> (w784:T2)
                n577 = local write "run lab01-1"(w783) -> ()
                n578 = case shown="True" w783 {
                  tunnel: w793 -> [_ w831]
                  tunnel: w792 -> [_ w830]
                  tunnel: w791 -> [w795 w829]
                  tunnel: w790 -> [_ w828]
                  tunnel: w789 -> [_ w827]
                  tunnel: [w794 w826] -> w788
                  tunnel: w787 -> [_ w825]
                  tunnel: w786 -> [_ w824]
                  tunnel: w785 -> [_ w823]
                  tunnel: w784 -> [_ w822]
                  tunnel: w782 -> [_ w821]
                  frame False {
                    # "stop test"
                    n579 = stacked-sequence {
                      tunnel: w795 -> [_ w807 _]
                      tunnel: [_ w799 _] -> w794
                      frame #0 {
                        n580 = local read "DISP LAB01-1"() -> (w798:T4)
                        n581 = Bundle(cluster=w798, "STATUS"="STOP") -> (w796:T4)  [unwired: 2 in]
                        n582 = local write "DISP LAB01-1"(w796) -> ()
                      }
                      frame #1 {
                        n583 = local read "DISP LAB01-1"() -> (w806:T4)
                        n584 = Unbundle(w806) -> ("CYCLE"=w804:dbl, "MINS"=w805:dbl)  [unwired: 1 out]
                        n585 = case shown="\"CYCLE TEST\"" w807 {
                          tunnel: w805 -> [_ _ w814]
                          tunnel: w804 -> [w812 w813 _]
                          tunnel: [w812 w813 w814] -> w803
                          frame "CHART TEST", Default {
                          }
                          frame "CYCLE TEST" {
                          }
                          frame "T-RISE TEST" {
                          }
                        }
                        n586 = local read "TDMS LAB01-1"() -> (w811:refnum<k34>)
                        n587 = Build Array("STOPPED") -> (w808:string[])
                        n588 = Build Array(w803) -> (w802:dbl[])
                        n589 = TDMS Write(0:w811, 5:"TEST RESULT", 7:w808, 9:w802) -> (4:w800:refnum<k34>, 15:w801:errorcluster)  [unwired: 2 in, 2 out]
                        n590 = TDMS Close(8:w801, 11:w800) -> (0:w799:errorcluster)  [unwired: 1 out]
                      }
                      frame #2 {
                        n591 = stacked-sequence {
                          tunnel: "LAB01-1" -> [w817 w819]
                          frame #0 {
                            n592 = call "sub vi - defrag tdms v1.vi"("panel id"=w817) -> ("error out"=w816:errorcluster)  [unwired: 10 in]
                            n593 = local write "data file error"(w816) -> ()
                          }
                          frame #1 {
                            n594 = call "Save data file (stop) v3.vi"("panel id"=w819) -> ("network file save error"=w818:errorcluster)  [unwired: 9 in, 1 out]
                            n595 = local write "RESULT LAB01-1"(FALSE) -> ()
                            n596 = local write "data file error"(w818) -> ()
                          }
                        }
                      }
                    }
                  }
                  frame True {
                    n597 = stacked-sequence {
                      seq-local: [w833 _] -> [_ w837]
                      tunnel: w831 -> [_ w847]
                      tunnel: w830 -> [_ w846]
                      tunnel: w829 -> [_ w845]
                      tunnel: w828 -> [_ w844]
                      tunnel: w827 -> [_ w843]
                      tunnel: [_ w842] -> w826
                      tunnel: w825 -> [_ w841]
                      tunnel: w824 -> [_ w840]
                      tunnel: w823 -> [_ w839]
                      tunnel: w822 -> [w835 w838]
                      tunnel: w821 -> [_ w836]
                      frame #0 {
                        n598 = Unbundle(w835) -> ("AMPS"=w834:dbl)  [unwired: 4 out]
                        n599 = call "Check For Amps on v1.vi"("ID"="LAB01-1", "amps"=w834) -> ("amps"=w833:bool)  [unwired: 9 in]
                      }
                      frame #1 {
                        n600 = case shown="True" w837 {
                          tunnel: w847 -> [_ w860]
                          tunnel: w846 -> [_ w859]
                          tunnel: w845 -> [_ w858]
                          tunnel: w844 -> [_ w857]
                          tunnel: w843 -> [_ w856]
                          tunnel: [errorcluster {"status"=FALSE, "code"=0, "source"=""} ("error out") w855] -> w842
                          tunnel: w841 -> [_ w854]
                          tunnel: w840 -> [_ w853]
                          tunnel: w839 -> [_ w852]
                          tunnel: w838 -> [_ w851]
                          tunnel: w836 -> [_ w850]
                          frame False {
                            w848 = FALSE
                            n601 = local write "RUN LAB01-1"(w848) -> ()
                            n602 = local write "run lab01-1"(w848) -> ()
                          }
                          frame True {
                            n603 = stacked-sequence {
                              seq-local: [w861 _ _ _ _] -> [_ w882 _ _ _]
                              tunnel: w860 -> [w866 _ _ _ _]
                              tunnel: w859 -> [w862 _ _ _ _]
                              tunnel: w858 -> [w876 _ _ _ _]
                              tunnel: w857 -> [w869 _ _ _ _]
                              tunnel: w856 -> [w864 _ _ _ _]
                              tunnel: [_ w883 _ _ _] -> w855
